vi "SQL Build Create Table Query.vi"(0 "data types":string[](array[string]), 1 "database":enum16{"dBase", "Jet", "SQL Server", "Oracle"}(ring), 2 "table":string, 3 "column information":T1[](array[typedef]), 4 "primary key (-1)":i32) -> (5 "字符串":string)   [LabVIEW 2011]
uses:
  <vilib>/addons/database/Auxilliary.llb/DB Tools Column Info.ctl
  <vilib>/addons/database/Auxilliary.llb/DB Tools DataTypes.ctl
  <vilib>/addons/database/NI_Database_API.lvlib
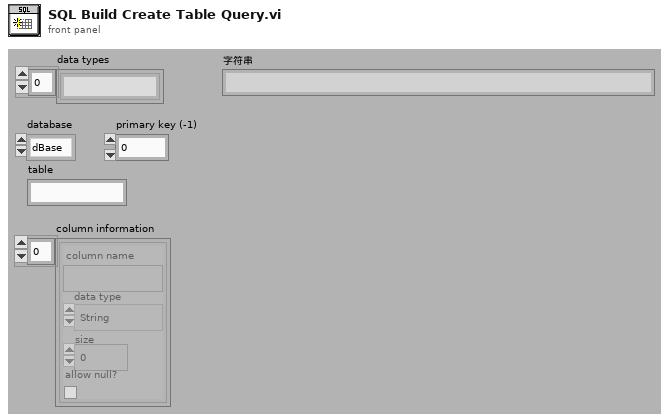
[diagram p1: front panel]
types:
  T1 = typedef "NI_Database_API.lvlib/DB Tools Column Info.ctl" = cluster{"column name":string, "data type":T2, "size":i32, "allow null?":bool}
  T2 = typedef "NI_Database_API.lvlib/DB Tools DataTypes.ctl" = enum16{"String", "Long (I32)", "Single (SGL)", "Double (DBL)", "Date/Time", "Binary"}
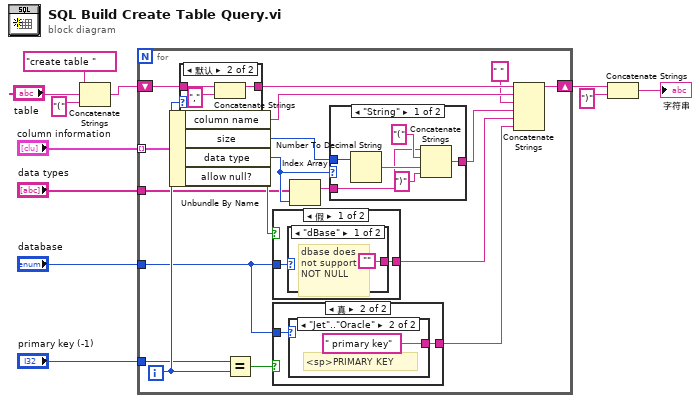
[diagram p0: block diagram]
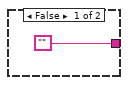
[diagram p2: hidden frame]
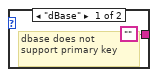
[diagram p3: hidden frame]
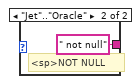
[diagram p4: hidden frame]
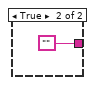
[diagram p5: hidden frame]
diagram:
  n1 = Concatenate Strings("create table " ("Substring"), "table", "(" ("Substring")) -> (w4:string)
  n2 = for {
    tunnel: "column information" -> [w29] mode=indexing
    shift-right: [w23] -> w5
    shift-left: w4 -> [w28]
    tunnel: "primary key (-1)" -> [w15]
    tunnel: "data types" -> [w13]
    tunnel: "database" -> [w12]
    i -> [w26]
    n3 = Unbundle By Name(w29) -> ("column name"=w21:string, "size"=w18:i32, "data type"=w19:T2, "allow null?"=w27:bool)
    n4 = case shown="默认" w26 {
      tunnel: [w47 w50] -> w22
      tunnel: w28 -> [w47 w48]
      frame 0 {
      }
      frame Default {
        n5 = Concatenate Strings(w48, "," ("Substring")) -> (w50:string)
      }
    }
    n6 = Equal?(x=w15, y=w26) -> (x = y?=w25:bool)
    n7 = case shown="假" w27 {
      tunnel: [w36 ""] -> w17
      tunnel: w12 -> [w35 _]
      frame False {
        n8 = case shown="\"dBase\"" w35 {
          tunnel: ["" " not null"] -> w36
          frame "dBase" {
            # "dbase does\nnot support\nNOT NULL"
          }
          frame "Jet".."Oracle" {
            # "<sp>NOT NULL"
          }
        }
      }
      frame True {
      }
    }
    n9 = case shown="真" w25 {
      tunnel: ["" w32] -> w16
      tunnel: w12 -> [_ w31]
      frame False {
      }
      frame True {
        n10 = case shown="\"Jet\"..\"Oracle\"" w31 {
          tunnel: ["" " primary key"] -> w32
          frame "dBase" {
            # "dbase does not \nsupport primary key"
          }
          frame "Jet".."Oracle" {
            # "<sp>PRIMARY KEY"
          }
        }
      }
    }
    n11 = Index Array(array=w13, index=w19) -> (element=w14:string)
    n12 = case shown="\"String\"" w19 {
      tunnel: w14 -> [w40 w46]
      tunnel: [w42 w46] -> w24
      tunnel: w18 -> [w41 _]
      frame "String" {
        n13 = Number To Decimal String(number=w41) -> (decimal integer string=w44:string)  [unwired: 1 in]
        n14 = Concatenate Strings(w40, "(" ("Substring"), w44, ")" ("Substring")) -> (w42:string)
      }
      frame "Long (I32)".."Binary" {
      }
    }
    n15 = Concatenate Strings(w22, w21, " " ("Substring"), w24, w17, w16) -> (w23:string)
  }
  n16 = Concatenate Strings(w5, ")" ("Substring")) -> (→"字符串":string)
